vi "angle_difference.vi"(1 "Angle 2":dbl, 2 "Angle 1":dbl) -> (0 "Difference":dbl)   [LabVIEW 2011]
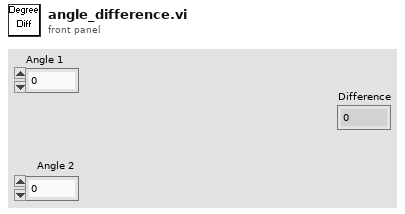
[diagram p1: front panel]
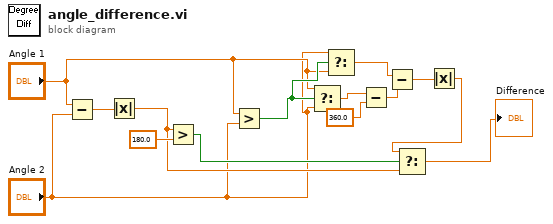
[diagram p0: block diagram]
diagram:
  n1 = Subtract(x="Angle 1", y="Angle 2") -> (x-y=w14:dbl)
  n2 = Absolute Value(x=w14) -> (abs(x)=w11:dbl)
  n3 = Greater?(x=w11, y=180.0) -> (0:w12:bool)
  n4 = Greater?(x="Angle 1", y="Angle 2") -> (0:w8:bool)
  n5 = Select(t="Angle 1", s=w8, f="Angle 2") -> (s? t:f=w10:dbl)
  n6 = Select(t="Angle 2", s=w8, f="Angle 1") -> (s? t:f=w3:dbl)
  n7 = Subtract(x=w10, y=360.0) -> (x-y=w4:dbl)
  n8 = Subtract(x=w3, y=w4) -> (x-y=w5:dbl)
  n9 = Absolute Value(x=w5) -> (abs(x)=w2:dbl)
  n10 = Select(t=w2, s=w12, f=w11) -> (s? t:f=→"Difference":dbl)
